vi "SG Filter (DVR).vi"(8 "error in":errorcluster, 10 "side points":i32, 11 "Data Value Reference in":refnum<data-value>) -> (0 "error out":errorcluster, 3 "Data Value Reference out":refnum<data-value>)   [LabVIEW 2016, in "Retrieve and Visualize.lvclass"]
uses:
  Retrieve and Visualize.lvclass
  <userlib>/LevyLab/XY Utilities/subVIs/Savitsky Golay Filter (multiple).vi
  <userlib>/LevyLab/XY Utilities/xy_utilities.lvlib
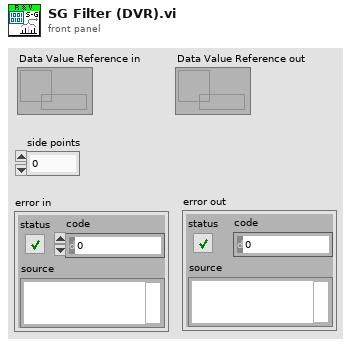
[diagram p1: front panel]
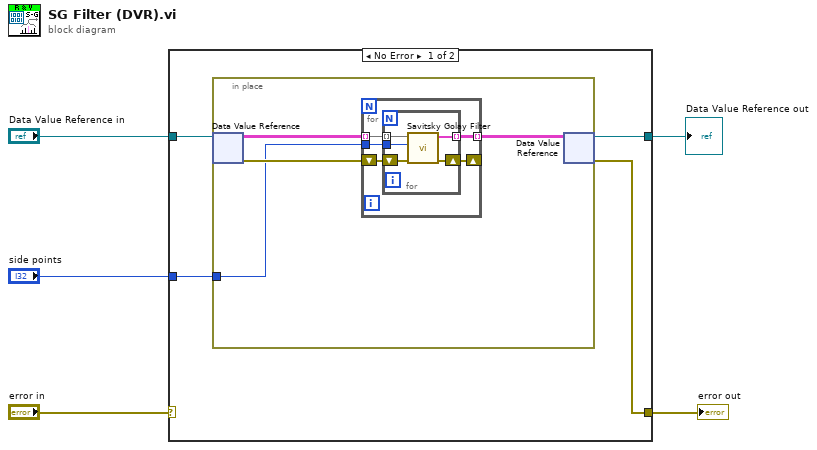
[diagram p0: block diagram]
diagram:
  n1 = case shown="No Error" "error in" {
    selector: "error in" -> [_ w25]
    tunnel: "side points" -> [w9 _]
    tunnel: [w8 w24] -> w4
    tunnel: "Data Value Reference in" -> [w7 w24]
    tunnel: [w6 w25] -> w2
    frame No Error {
      n2 = in-place {
        in-place-border: w9 -> [w10]
        n3 = in-place-dvr #1(w7) -> (w13:cluster{dbl[], dbl[]}[][][], w11:errorcluster)
        n4 = for {
          tunnel: [w18] -> w12 mode=indexing
          tunnel: w10 -> [w17]
          tunnel: w13 -> [w16] mode=indexing
          shift-right: [w14] -> _
          shift-left: w11 -> [w15]
          n5 = for {
            tunnel: [w22] -> w18 mode=indexing
            tunnel: w17 -> [w23]
            tunnel: w16 -> [w21] mode=indexing
            shift-right: [w19] -> w14
            shift-left: w15 -> [w20]
            n6 = call-poly <userlib>:"Savitsky Golay Filter.vi"("error in (no error)"=w20, "side points"=w23, "XY-data"=w21) -> ("error out"=w19:errorcluster, "XY-data out"=w22:cluster{"X-array":dbl[], "Y-array":dbl[]}[])  [unwired: 7 in]
          }
        }
        n7 = in-place-dvr #1(w12) -> (w8:refnum<data-value>, w6:errorcluster)
      }
    }
    frame Error {
    }
  }
  "Data Value Reference out" <- w4
  "error out" <- w2
